vi "auto_ctrl_thcd401_ch1.vi"(4 "ref_reinit":refnum<vi>, 6 "ref_sp_ch1":refnum<vi>, 7 "time_last_ctrl_in":timestamp, 8 "flow_params":dbl[](array[numeric]) format="%#_13g", 9 "P_set":dbl=1.0 format="%#_13g", 10 "enable_auto_ctrl":bool caption="Auto Control", 11 "ref_magnet_pres":refnum<vi>) -> (0 "F_new":dbl format="%.3f", 1 "status":u32(colorbox), 2 "P_psi":dbl=1.1 format="%.2f", 3 "P_Torr":dbl=1.1 format="%.1f", 5 "time_last_ctrl_out":timestamp)   [LabVIEW 2019]
doc: "This example demonstrates how to simulate a general PID controller."
uses:
  <vilib>/addons/control/pid/pid.llb/PID (DBL).vi
  <vilib>/addons/control/pid/NI_PID_pid.lvlib
panel:
  out "MV":dbl format="%.1f"
  in  "ctrl_interval":dbl=0.5
  in  "P_max":dbl=1.4 format="%.1f"
  in  "P_min":dbl=-0.4 format="%.1f"
  in  "PID Range":cluster{"High":dbl, "Low":dbl}={"High"=20.0, "Low"=-20.0} {"Low" format="%.1f"; "High" format="%.1f"}
  in  "PID gains":T1={"proportional gain (Kc)"=-17.0, "integral time (Ti, min)"=0.2, "derivative time (Td, min)"=0.1} {"derivative time (Td, min)" format="%.4f"; "integral time (Ti, min)" format="%.4f"; "proportional gain (Kc)" format="%.3f"}
  # "sec"
  # "psi"
  # "psi"
  # "flow_min"
  # "flow_max"
  # "flow_org"
  # "L/m"
  # "L/m"
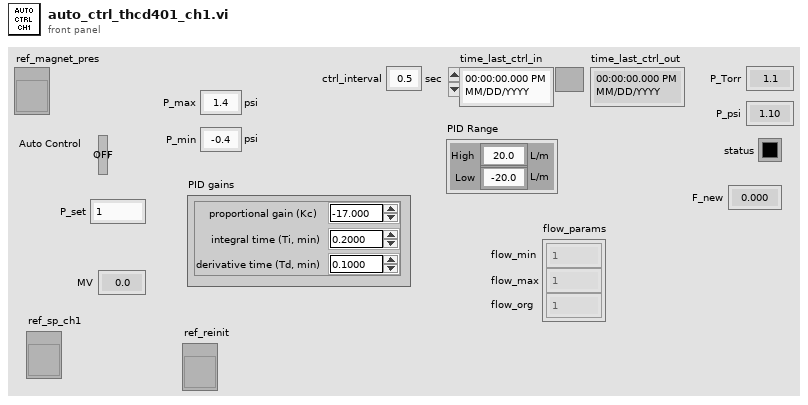
[diagram p1: front panel]
types:
  T1 = cluster{"proportional gain (Kc)":dbl, "integral time (Ti, min)":dbl, "derivative time (Td, min)":dbl}
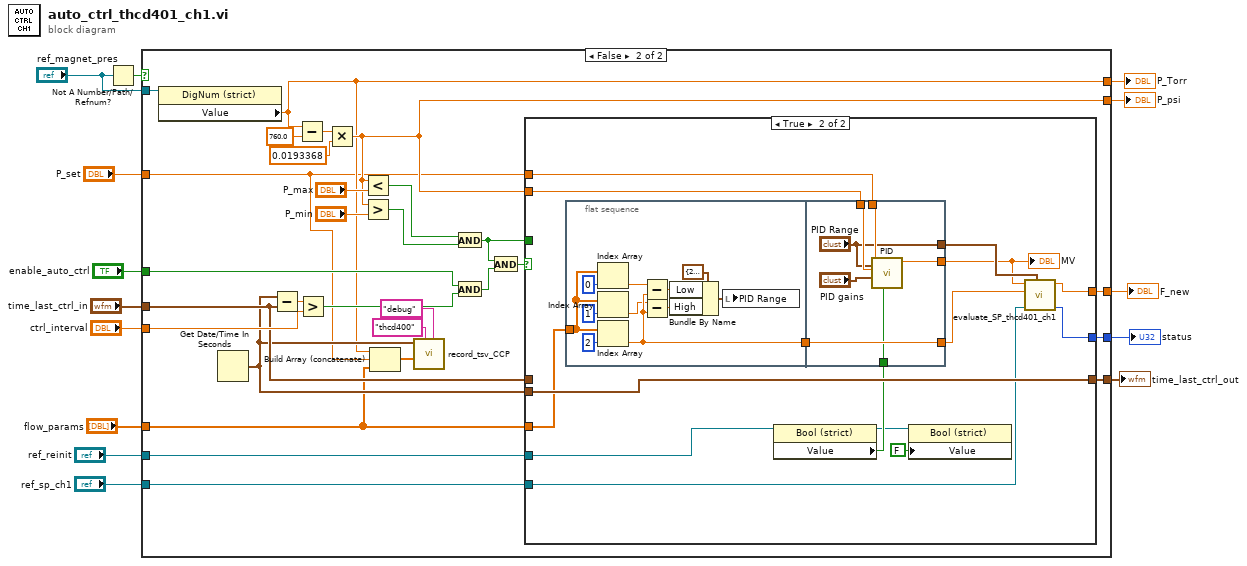
[diagram p0: block diagram]
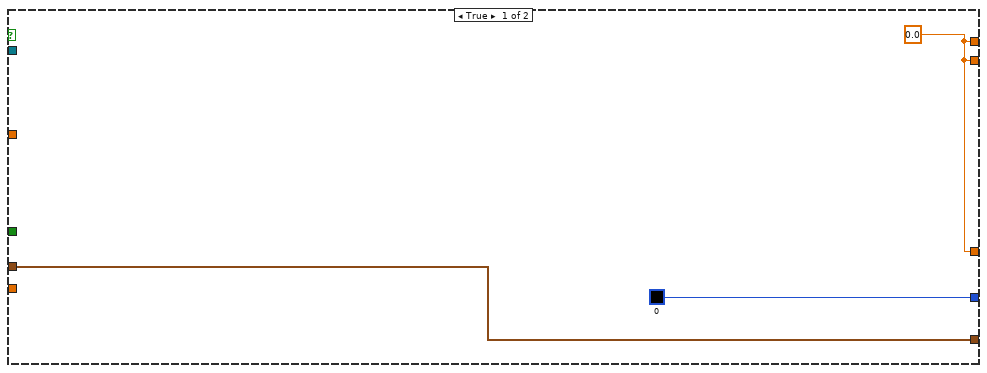
[diagram p2: hidden frame]
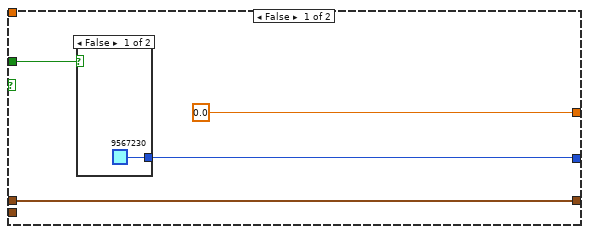
[diagram p3: hidden frame]
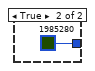
[diagram p4: hidden frame]
diagram:
  n1 = Not A Number/Path/Refnum?(number/path/refnum="ref_magnet_pres") -> (NaN/Path/Refnum?=w10:bool)
  n2 = case shown="False" w10 {
    tunnel: "ref_magnet_pres" -> [_ w44]
    tunnel: [w17 w46] -> w13
    tunnel: [u32 0 ("alarm_status") w45] -> w12
    tunnel: "P_set" -> [_ w20]
    tunnel: "enable_auto_ctrl" -> [_ w29]
    tunnel: [w17 w21] -> w8
    tunnel: [w17 w38] -> w7
    tunnel: "ref_sp_ch1" -> [_ w37]
    tunnel: "time_last_ctrl_in" -> [w15 w33]
    tunnel: "ctrl_interval" -> [_ w35]
    tunnel: [w15 w34] -> w3
    tunnel: "flow_params" -> [_ w19]
    tunnel: "ref_reinit" -> [_ w25]
    frame True {
      w17 = 0.0 ("Value")
    }
    frame False {
      n3 = property on="Property Node" class="DigNum (strict)"(reference=w44) -> ("Value"=w21:dbl)  [unwired: 1 in, 2 out]
      n4 = Get Date/Time In Seconds() -> (seconds since 1Jan1904=w22:timestamp)
      n5 = Subtract(x=w22, y=w33) -> (x-y=w36:dbl)
      n6 = Subtract(x=w21, y=760.0) -> (x-y=w42:dbl)
      n7 = Greater?(x=w36, y=w35) -> (0:w30:bool)
      n8 = Multiply(x=w42, y=0.0193368) -> (x*y=w38:dbl)
      n9 = Less?(x=w38, y="P_max") -> (x < y?=w27:bool)
      n10 = Greater?(x=w38, y="P_min") -> (0:w28:bool)
      n11 = Build Array (concatenate)(w21, w20, w19) -> (w18:dbl[])
      n12 = call "record_tsv_CCP.vi"("file_name"="debug", "folder_name"="thcd400", "value_array"=w18, "time"=w22) -> ()  [unwired: 6 in, 2 out]
      n13 = And(x=w27, y=w28) -> (x .and. y?=w26:bool)
      n14 = And(x=w29, y=w30) -> (x .and. y?=w31:bool)
      n15 = And(x=w26, y=w31) -> (x .and. y?=w32:bool)
      n16 = case shown="True" w32 {
        tunnel: [0.0 ("F_O_new") w64] -> w46
        tunnel: [w47 w67] -> w45
        tunnel: w20 -> [_ w59]
        tunnel: w38 -> [_ w60]
        tunnel: w37 -> [_ w65]
        tunnel: [w49 w66] -> w34
        tunnel: w22 -> [_ w66]
        tunnel: w33 -> [w49 _]
        tunnel: w26 -> [w48 _]
        tunnel: w19 -> [_ w63]
        tunnel: w25 -> [_ w56]
        frame False {
          n17 = case shown="False" w48 {
            tunnel: [u32 9567230 ("alarm_status") u32 1985280 ("alarm_status")] -> w47
            frame False {
            }
            frame True {
            }
          }
        }
        frame True {
          n18 = flat-sequence {
            tunnel: w63 -> [w75]
            tunnel: [w70] -> w61
            tunnel: [w85] -> w62
            tunnel: w61 -> [w85]
            tunnel: w60 -> [w83]
            tunnel: w59 -> [w82]
            tunnel: ["PID Range"] -> w58
            tunnel: [w80] -> w57
            tunnel: w55 -> [w79]
            frame #0 {
              n19 = Index Array(array=w75, index=0) -> (element=w69:dbl)
              n20 = Index Array(array=w75, index=1) -> (element=w68:dbl)
              n21 = Index Array(array=w75, index=2) -> (element=w70:dbl)
              n22 = Subtract(x=w69, y=w70) -> (x-y=w71:dbl)
              n23 = Subtract(x=w68, y=w70) -> (x-y=w72:dbl)
              n24 = Bundle By Name(cluster=cluster{"High":dbl, "Low":dbl} {"High"=20.0, "Low"=-20.0} ("PID Range"), "Low"=w71, "High"=w72) -> (w74:cluster{"High":dbl, "Low":dbl})
              n25 = local write "PID Range"(w74) -> ()
            }
            frame #1 {
              n26 = call-poly <vilib>:"PID.vi"("reinitialize? (F)"=w79, "output range"="PID Range", "PID gains"="PID gains", "process variable"=w83, "setpoint"=w82) -> ("output"=w80:dbl)  [unwired: 5 in, 1 out]
            }
          }
          n27 = property class="Bool (strict)"(reference=w56) -> (reference out=w54:refnum<vi>, "Value"=w55:bool)  [unwired: 1 in, 1 out]
          n28 = property class="Bool (strict)"(reference=w54, "Value"=FALSE) -> ()  [unwired: 1 in, 2 out]
          n29 = call "evaluate_SP_thcd401_ch1.vi"("PID Range"=w58, "ref_sp_ch1"=w65, "F_org"=w62, "control"=w57) -> ("status"=w67:u32, "F_new"=w64:dbl)  [unwired: 6 in]
          "MV" <- w57
        }
      }
    }
  }
  "F_new" <- w13
  "status" <- w12
  "P_Torr" <- w8
  "P_psi" <- w7
  "time_last_ctrl_out" <- w3
